vi "Main VI.vi"() -> ()   [LabVIEW 2017]
uses:
  I28 Drivers/I28Drivers.lvlib
panel:
  out "Timeout Message":string
  in  "Send Command":bool
  in  "Enter Command":string
  out "Connected to I28?":bool
  in  "Start Test":bool
  in  "stop":bool
  out "Raw Data":string
  in  "Turn On Results":bool
  out "Currently Active Program":string
  in  "Get CAP":bool
  out "ErrorOut":errorcluster
  out "Result Data":string
  # "Debugging Controls and Indicators"
  # "1.M\\S1TCAP - Read CAP\n2.M\\S1TCAP=# - Changes CAP"
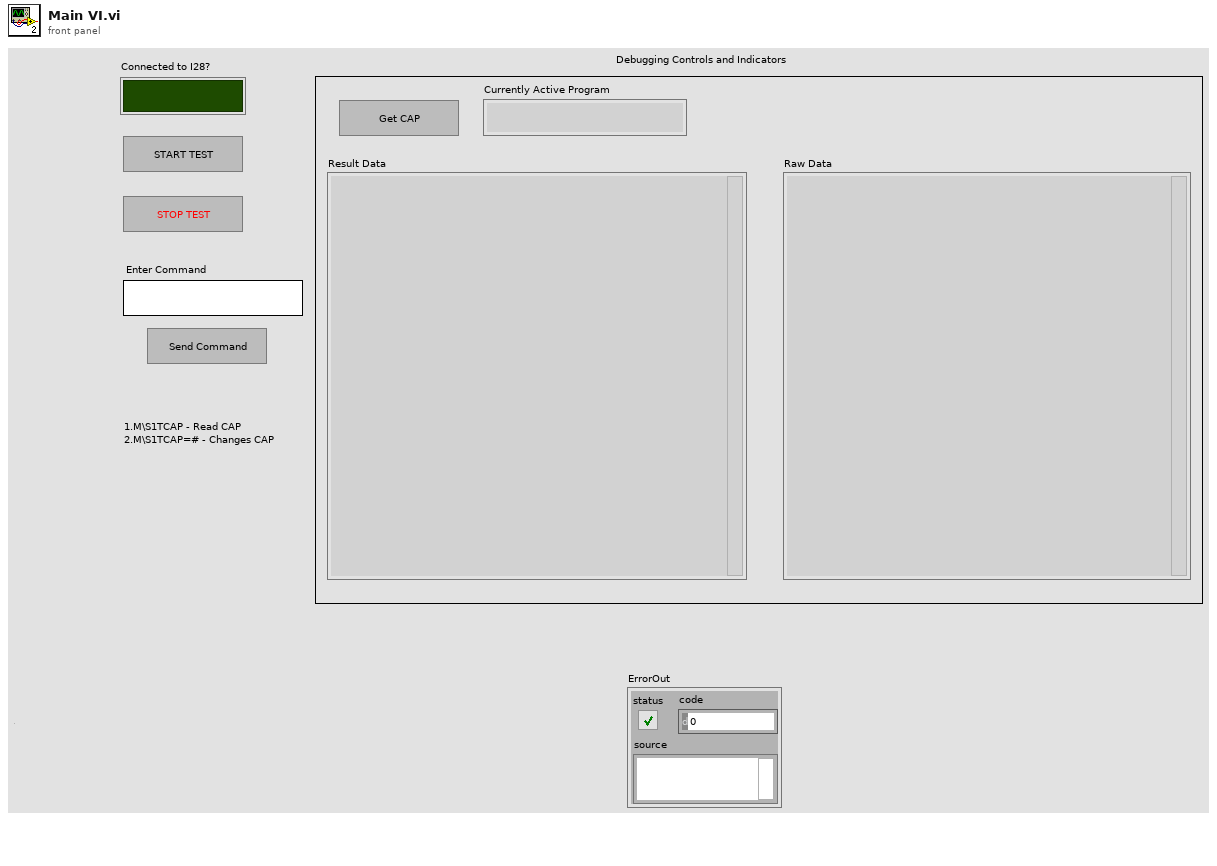
[diagram p1: front panel]
types:
  T1 = enum8{"Enabled", "Disabled", "Disabled and Grayed Out"}
  T2 = enum16{"open", "replace", "create", "open or create", "replace or create", "replace or create with confirmation"}
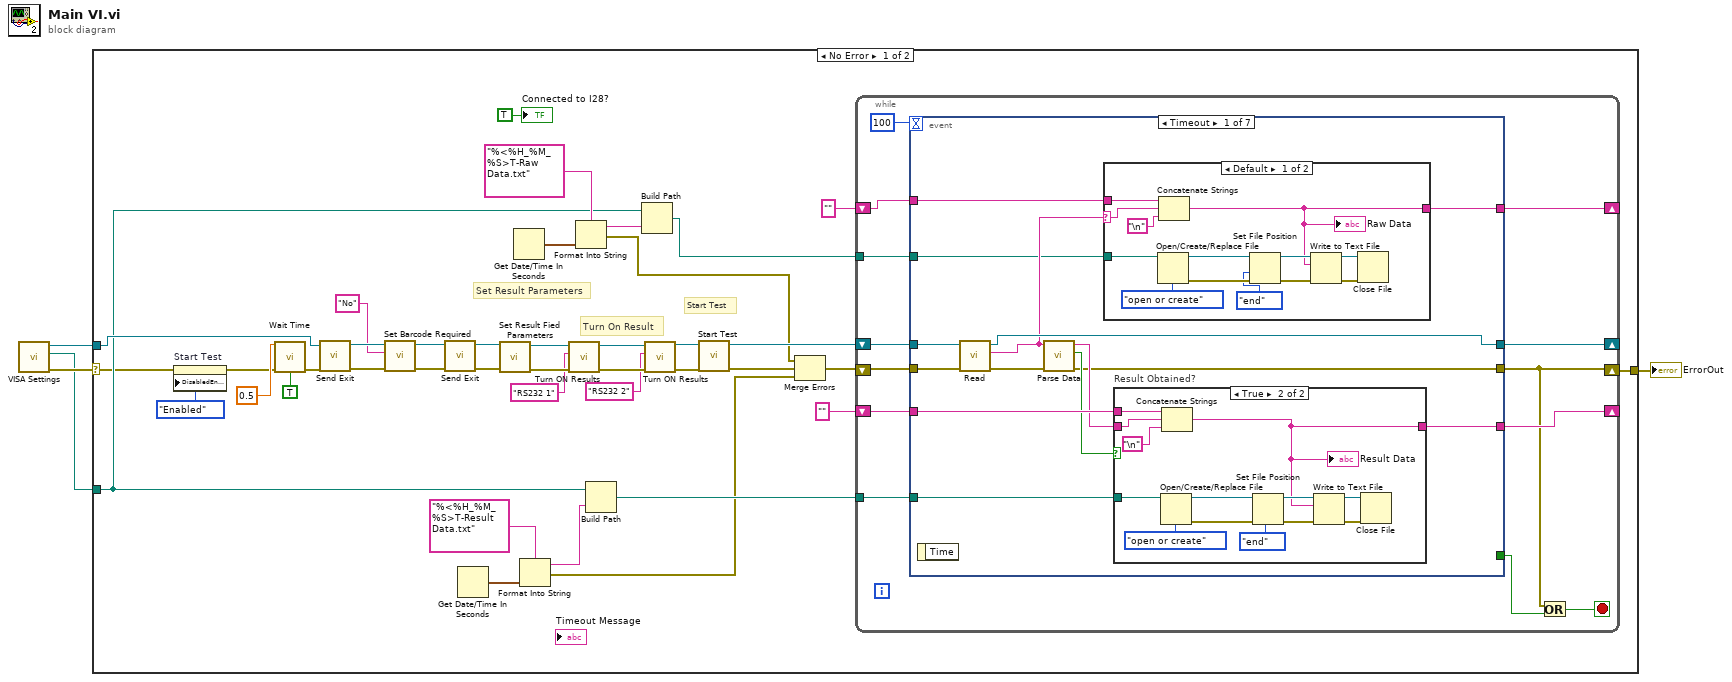
[diagram p0: block diagram]
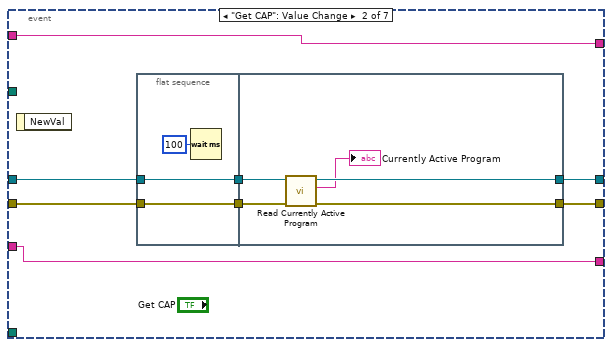
[diagram p4: hidden frame]
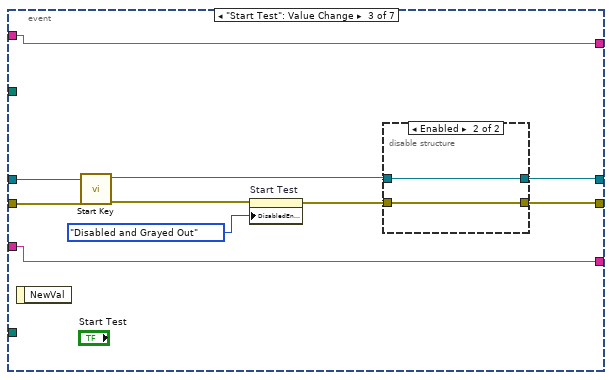
[diagram p5: hidden frame]
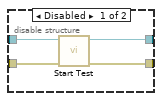
[diagram p6: hidden frame]
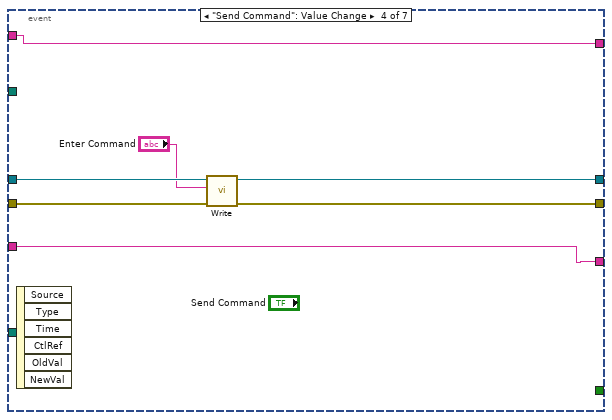
[diagram p7: hidden frame]
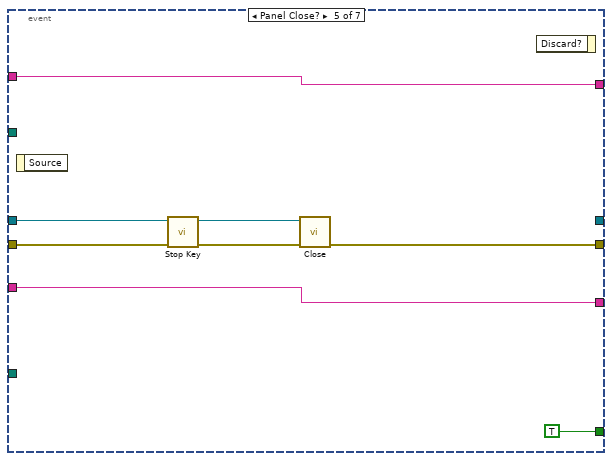
[diagram p8: hidden frame]
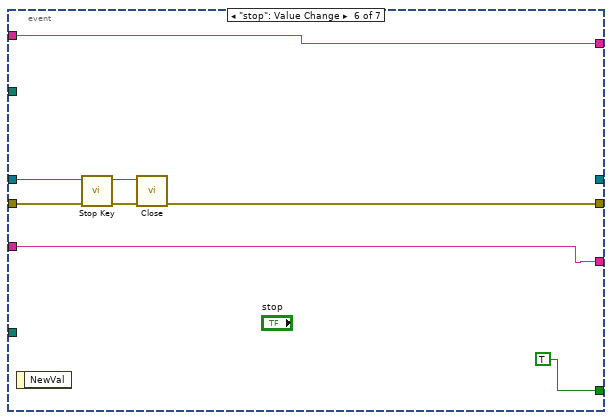
[diagram p9: hidden frame]
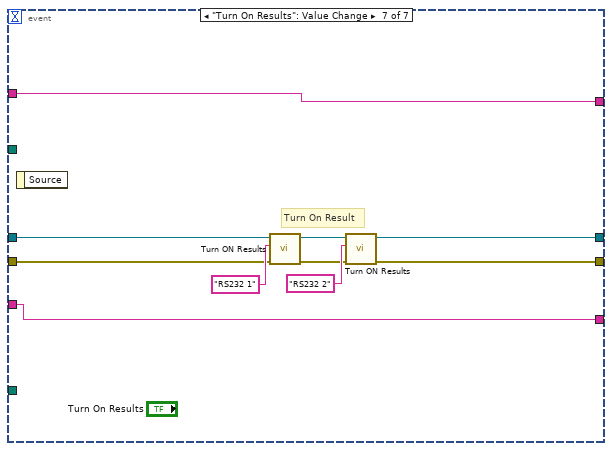
[diagram p10: hidden frame]
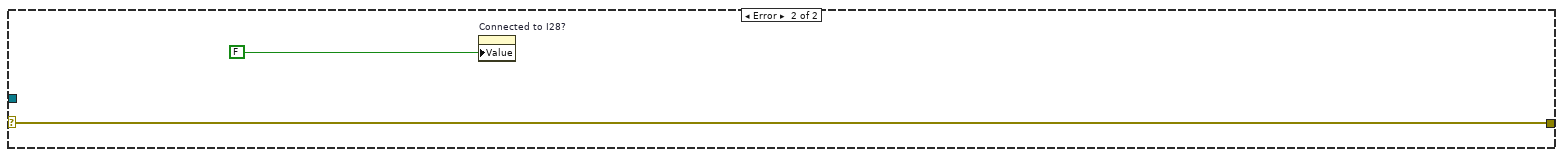
[diagram p11: hidden frame]
diagram:
  n1 = call "VISA Settings.vi"() -> ("ErrorOut"=w4:errorcluster, "Path Out"=w1:path, "VISA resource name out"=w3:refnum<visa-resource-name>)  [unwired: 9 in]
  n2 = case shown="No Error" w4 {
    selector: w4 -> [w19 w166]
    tunnel: w3 -> [w44 _]
    tunnel: [w33 w166] -> w2
    tunnel: w1 -> [w22 _]
    frame No Error {
      # "Set Result Parameters"
      # "Start Test"
      # "Turn On Result"
      n3 = property on="Start Test" class="Bool"(error in=w19, "DisabledEnum"=T1."Enabled" ("Disabled")) -> (error out=w10:errorcluster)  [unwired: 1 in, 1 out]
      n4 = call "Wait Time.vi"("Delay Time (s)"=0.5, "error in"=w10, "Set Time"=TRUE) -> ("error out"=w9:errorcluster)  [unwired: 12 in]
      n5 = call "Send Exit.vi"("ErrorIn"=w9, "VISAIn"=w44) -> ("ErrorOut"=w17:errorcluster, "VISAOut"=w16:refnum<visa-resource-name>)  [unwired: 7 in, 1 out]
      n6 = call "Set Barcode Required.vi"("ErrorIn"=w17, "Command"="No", "VISAIn"=w16) -> ("ErrorOut"=w15:errorcluster, "VISAOut"=w14:refnum<visa-resource-name>)  [unwired: 7 in]
      n7 = call "Send Exit.vi"("ErrorIn"=w15, "VISAIn"=w14) -> ("ErrorOut"=w11:errorcluster, "VISAOut"=w13:refnum<visa-resource-name>)  [unwired: 7 in, 1 out]
      n8 = Get Date/Time In Seconds() -> (seconds since 1Jan1904=w30:timestamp)
      n9 = call "Set Result Fied Parameters.vi"("ErrorIn"=w11, "VISAIn"=w13) -> ("ErrorOut"=w42:errorcluster, "VISAOut"=w43:refnum<visa-resource-name>)  [unwired: 8 in]
      n10 = Get Date/Time In Seconds() -> (seconds since 1Jan1904=w23:timestamp)
      n11 = Format Into String(format string="%<%H_%M_%S>T-Result Data.txt", w30) -> (resulting string=w28:string, error out=w6:errorcluster)  [unwired: 2 in]
      n12 = call "Turn ON Results.vi"("ErrorIn"=w42, "Command"="RS232 1", "VISAIn"=w43) -> ("ErrorOut"=w41:errorcluster, "VISAOut"=w40:refnum<visa-resource-name>)  [unwired: 6 in, 1 out]
      n13 = Format Into String(format string="%<%H_%M_%S>T-Raw Data.txt", w23) -> (resulting string=w25:string, error out=w5:errorcluster)  [unwired: 2 in]
      n14 = Build Path(base path=w22, name or relative path=w28) -> (appended path=w27:path)
      n15 = Build Path(base path=w22, name or relative path=w25) -> (appended path=w21:path)
      n16 = call "Turn ON Results.vi"("ErrorIn"=w41, "Command"="RS232 2", "VISAIn"=w40) -> ("ErrorOut"=w37:errorcluster, "VISAOut"=w36:refnum<visa-resource-name>)  [unwired: 6 in, 1 out]
      n17 = call "Start Test.vi"("ErrorIn"=w37, "VISAIn"=w36) -> ("ErrorOut"=w8:errorcluster, "VISAOut"=w35:refnum<visa-resource-name>)  [unwired: 7 in, 1 out]
      n18 = Merge Errors(w5, w8, w6) -> (w7:errorcluster)
      n19 = while {
        shift-right: [w53] -> _
        shift-left: w35 -> [w54]
        shift-right: [w51] -> _
        shift-left: "" -> [w52]
        shift-right: [w49] -> w33
        shift-left: w7 -> [w56]
        tunnel: w27 -> [w48]
        shift-right: [w46] -> _
        shift-left: "" -> [w47]
        tunnel: w21 -> [w45]
        stop <- w50 stop-if-true
        n20 = event shown="[0] Timeout" {
          selector: _ -> [_ _ _ _ _ _ _]
          dyn-events: _ -> [_ _ _ _ _ _ _]
          timeout: 100 -> [_ _ _ _ _ _ _]
          tunnel: w56 -> [w71 w105 w124 w136 w142 w150 w160]
          tunnel: [_ _ _ _ TRUE TRUE _] -> w55
          tunnel: w54 -> [w70 w107 w123 w134 w140 w148 w159]
          tunnel: [w64 w106 w116 w133 _ _ w157] -> w53
          tunnel: w52 -> [w68 w103 w125 w138 w145 w153 w156]
          tunnel: [w65 w103 w125 w138 w145 w153 w156] -> w51
          tunnel: [w63 w104 w118 w135 w144 w151 w158] -> w49
          tunnel: w48 -> [w62 _ _ _ _ _ _]
          tunnel: w47 -> [w60 w102 w122 w137 w143 w154 w155]
          tunnel: [w59 w102 w122 w137 w143 w154 w155] -> w46
          tunnel: w45 -> [w58 _ _ _ _ _ _]
          event Timeout {
            n21 = event-data() -> ()  [unwired: 1 in, 1 out]
            n22 = call "Read.vi"("ErrorIn"=w71, "VISAIn"=w70) -> ("ErrorOut"=w69:errorcluster, "Data"=w61:string, "VISAOut"=w64:refnum<visa-resource-name>)  [unwired: 7 in]
            n23 = call "Parse Data.vi"("error in"=w69, "Data In"=w61) -> ("error out"=w63:errorcluster, "Result?"=w66:bool, "Result Data Out"=w67:string)  [unwired: 7 in]
            n24 = case shown="Default" w61 {
              selector: w61 -> [w83 _]
              tunnel: w60 -> [w84 w85]
              tunnel: [w73 w85] -> w59
              tunnel: w58 -> [w74 _]
              frame Default {
                n25 = Open/Create/Replace File(file path (use dialog)=w74, operation (0:open)=T2."open or create") -> (refnum out=w77:refnum<file>, error out=w78:errorcluster)  [unwired: 4 in, 1 out]
                n26 = Concatenate Strings(w84, w83, "\n") -> (w73:string)
                "Raw Data" <- w73
                n27 = Set File Position(refnum=w77, from (0:start)=enum16{"start", "end", "current"}."end", error in=w78) -> (refnum out=w81:refnum<file>, error out=w80:errorcluster)  [unwired: 1 in]
                n28 = Write to Text File(file (use dialog)=w81, text=w73, error in=w80) -> (refnum out=w75:refnum<file>, error out=w76:errorcluster)  [unwired: 1 in, 1 out]
                n29 = Close File(refnum=w75, error in=w76) -> ()  [unwired: 2 out]
              }
              frame "" {
              }
            }
            n30 = case "Result Obtained?" shown="True" w66 {
              tunnel: w68 -> [w86 w99]
              tunnel: w67 -> [_ w87]
              tunnel: [w86 w94] -> w65
              tunnel: w62 -> [_ w90]
              frame False {
              }
              frame True {
                n31 = Open/Create/Replace File(file path (use dialog)=w90, operation (0:open)=T2."open or create") -> (refnum out=w91:refnum<file>, error out=w92:errorcluster)  [unwired: 4 in, 1 out]
                n32 = Concatenate Strings(w99, w87, "\n") -> (w94:string)
                "Result Data" <- w94
                n33 = Set File Position(refnum=w91, from (0:start)=enum16{"start", "end", "current"}."end", error in=w92) -> (refnum out=w97:refnum<file>, error out=w96:errorcluster)  [unwired: 1 in]
                n34 = Write to Text File(file (use dialog)=w97, text=w94, error in=w96) -> (refnum out=w88:refnum<file>, error out=w89:errorcluster)  [unwired: 1 in, 1 out]
                n35 = Close File(refnum=w88, error in=w89) -> ()  [unwired: 2 out]
              }
            }
          }
          event "Get CAP": Value Change {
            n36 = event-data() -> ()  [unwired: 1 in, 1 out]
            n37 = flat-sequence {
              tunnel: w105 -> [w109]
              tunnel: w107 -> [w110]
              tunnel: [w110] -> w101
              tunnel: [w109] -> w100
              tunnel: [w114] -> w106
              tunnel: [w112] -> w104
              tunnel: w101 -> [w115]
              tunnel: w100 -> [w113]
              frame #0 {
                n38 = Wait (ms)(milliseconds to wait=u32 100) -> ()  [unwired: 1 out]
              }
              frame #1 {
                n39 = call "Read Currently Active Program.vi"("ErrorIn"=w113, "VISAIn"=w115) -> ("ErrorOut"=w112:errorcluster, "Data"=→"Currently Active Program":string, "VISAOut"=w114:refnum<visa-resource-name>)  [unwired: 7 in]
              }
            }
          }
          event "Start Test": Value Change {
            n40 = event-data() -> ()  [unwired: 1 in, 1 out]
            n41 = call "Start Key.vi"("ErrorIn"=w124, "VISAIn"=w123) -> ("ErrorOut"=w120:errorcluster, "VISAOut"=w117:refnum<visa-resource-name>)  [unwired: 8 in]
            n42 = property on="Start Test" class="Bool"(error in=w120, "DisabledEnum"=T1."Disabled and Grayed Out" ("Disabled")) -> (error out=w119:errorcluster)  [unwired: 1 in, 1 out]
            n43 = disable-structure shown="Enabled" {
              disable-tunnel: w119 -> [w129 w130]
              disable-tunnel: [w128 w130] -> w118
              disable-tunnel: w117 -> [w127 w131]
              disable-tunnel: [w126 w131] -> w116
              frame Disabled {
                n44 = call "Start Test.vi"("ErrorIn"=w129, "VISAIn"=w127) -> ("ErrorOut"=w128:errorcluster, "VISAOut"=w126:refnum<visa-resource-name>)  [unwired: 7 in, 1 out]
              }
              frame Enabled {
              }
            }
          }
          event "Send Command": Value Change {
            n45 = event-data() -> ()  [unwired: 1 in, 6 out]
            n46 = call "Write.vi"("ErrorIn"=w136, "Command"="Enter Command", "VISAIn"=w134) -> ("ErrorOut"=w135:errorcluster, "VISAOut"=w133:refnum<visa-resource-name>)  [unwired: 7 in]
          }
          event Panel Close? {
            n47 = event-data() -> ()  [unwired: 1 in, 1 out]
            n48 = call "Stop Key.vi"("ErrorIn"=w142, "VISAIn"=w140) -> ("ErrorOut"=w141:errorcluster, "VISAOut"=w139:refnum<visa-resource-name>)  [unwired: 8 in]
            n49 = call "Close.vi"("ErrorIn"=w141, "VISAIn"=w139) -> ("ErrorOut"=w144:errorcluster)  [unwired: 9 in]
            n50 = event-data() -> ()  [unwired: 2 in, 1 out]
          }
          event "stop": Value Change {
            n51 = event-data() -> ()  [unwired: 1 in, 1 out]
            n52 = call "Stop Key.vi"("ErrorIn"=w150, "VISAIn"=w148) -> ("ErrorOut"=w149:errorcluster, "VISAOut"=w147:refnum<visa-resource-name>)  [unwired: 8 in]
            n53 = call "Close.vi"("ErrorIn"=w149, "VISAIn"=w147) -> ("ErrorOut"=w151:errorcluster)  [unwired: 9 in]
          }
          event "Turn On Results": Value Change {
            # "Turn On Result"
            n54 = event-data() -> ()  [unwired: 1 in, 1 out]
            n55 = call "Turn ON Results.vi"("ErrorIn"=w160, "Command"="RS232 1", "VISAIn"=w159) -> ("ErrorOut"=w161:errorcluster, "VISAOut"=w162:refnum<visa-resource-name>)  [unwired: 6 in, 1 out]
            n56 = call "Turn ON Results.vi"("ErrorIn"=w161, "Command"="RS232 2", "VISAIn"=w162) -> ("ErrorOut"=w158:errorcluster, "VISAOut"=w157:refnum<visa-resource-name>)  [unwired: 6 in, 1 out]
          }
        }
        n57 = Or(x=w49, y=w55) -> (x .or. y?=w50:bool)
      }
      "Connected to I28?" <- TRUE ("Connected to I28?")
    }
    frame Error {
      n58 = property on="Connected to I28?" class="Bool (strict)"("Value"=FALSE ("Connected to I28?")) -> ()  [unwired: 2 in, 2 out]
    }
  }
  "ErrorOut" <- w2
